vi "dfd_Get NStage VI Description.vi"(6 "nStage nMAC Parameters":T1[](array[typedef]), 7 "multirate filters":T6[](array[typedef]) {"mMRate_SumWl" min=1 max=32 step=1; "mMRate_InputIwl" min=1 max=32 step=1; "mMRate_GainWl" min=1 max=32 step=1; "mMRate_OutputWl" min=1 max=32 step=1; "mMRate_InputWl" min=1 max=32 step=1; "mMRate_CoefWl" min=1 max=32 step=1; "mMRate_Mode" items=["Default"=-1, "No Rate Change"=0, "Interpolation"=1, "Decimation"=2, "Interpolated"=3, "Rational"=4]}, 8 "error in (no error)":errorcluster, 9 "feedback string":string[](array[string]), 10 "M":i32, 11 "L":i32) -> (0 "error out":errorcluster, 3 "NStage VI description":string)   [LabVIEW 2017, in "NI_DigFilterLicensed.lvlib"]
uses:
  <vilib>/addons/Digital Filter Design/NI_DigFilterLicensed.lvlib
  <vilib>/addons/Digital Filter Design/_Objects.llb/DFD Multirate Filter Obj.ctl
  <vilib>/addons/Digital Filter Design/_Objects.llb/DFD Multirate Mode.ctl
  <vilib>/addons/Digital Filter Design/_Objects.llb/DFD Coef Norm Type.ctl
  <vilib>/addons/Digital Filter Design/_Objects.llb/DFD Round-off Mode.ctl
  <vilib>/addons/Digital Filter Design/_Objects.llb/DFD FXP MRate Multiply Mode.ctl
  <vilib>/addons/Digital Filter Design/nMAC.llb/Typedefs/dfd_nMAC_Implementation Parameter.ctl
  <vilib>/addons/Digital Filter Design/nMAC.llb/Typedefs/dfd_nMAC_Execution Mode.ctl
  <vilib>/addons/Digital Filter Design/nMAC.llb/Typedefs/dfd_nMAC_Memory Type.ctl
  <vilib>/addons/Digital Filter Design/nMAC.llb/Typedefs/dfd_nMAC_Coef Reload API.ctl
  <vilib>/addons/Digital Filter Design/nMAC.llb/Typedefs/dfd_nMAC_Coef Map Type.ctl
  <vilib>/addons/Digital Filter Design/NI_DigFilter_CodeGen.lvlib
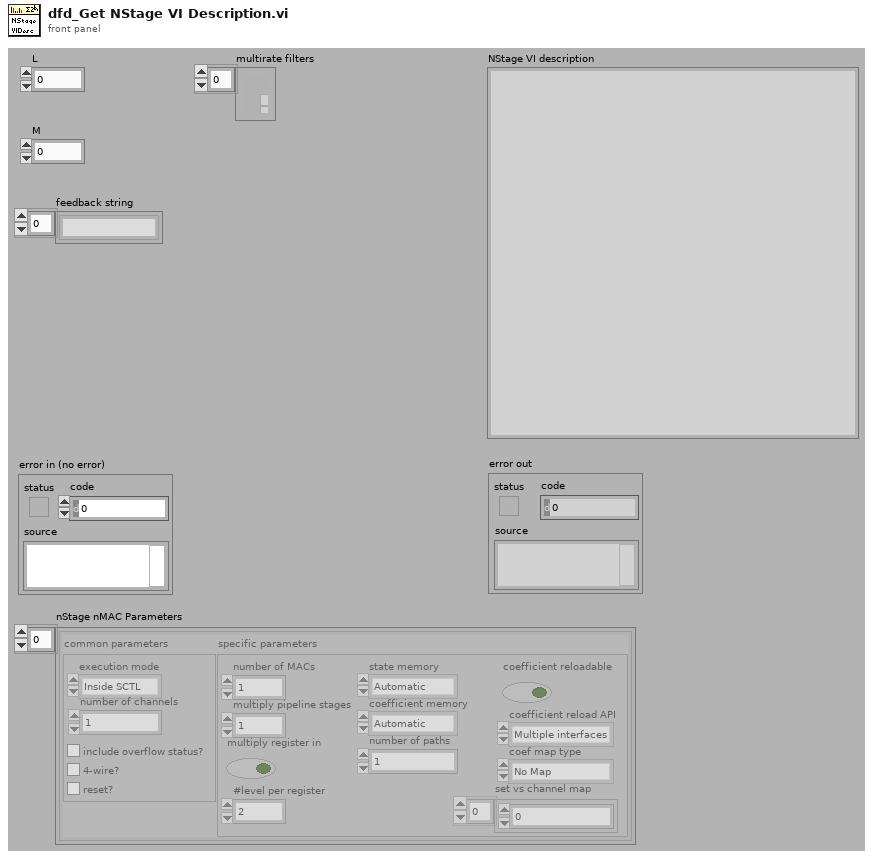
[diagram p1: front panel]
types:
  T1 = typedef "dfd_nMAC_Implementation Parameter.ctl" = cluster{"common parameters":cluster{"execution mode":T2, "number of channels":u32, "reset":bool, "include overflow status":bool, "4-wire":bool}, "specific parameters":cluster{"number of MACs":u32, "multiply pipeline stages":u32, "multiply register in":bool, "#level per register":u32, "state memory":T3, "coefficient memory":T3, "number of paths":u32, "coefficient reloadable":bool, "coefficient reload API":T4, "coef map type":T5, "set vs channel map":u32[]}}
  T2 = typedef "dfd_nMAC_Execution Mode.ctl" = enum16{"Outside SCTL", "Inside SCTL"}
  T3 = typedef "dfd_nMAC_Memory Type.ctl" = enum16{"Automatic", "BRAM", "DRAM"}
  T4 = typedef "dfd_nMAC_Coef Reload API.ctl" = enum16{"Multiple interfaces", "Single interface"}
  T5 = typedef "dfd_nMAC_Coef Map Type.ctl" = enum16{"No Map", "Set Map", "Channel Map"}
  T6 = typedef "NI_DigFilterLicensed.lvlib/DFD Multirate Filter Obj.ctl" = cluster{"mMRate_Structure":enum16{"CIC", "FIR", "IIR", "Lattice"}, "mMRate_Mode":T7, "mMRate_Factor":i32, "mMRate_FIRParams":cluster{"mMRate_FIR_H":dbl[], "mMRate_FIR_IsNyquist?":bool, "mMRate_FIR_IsSymmetric?":bool}, "mMRate_CICParams":cluster{"mMRate_CIC_#Stage":i32, "mMRate_CIC_Lag":i32, "mMRate_CIC_Type":enum16{"Lowpass", "Highpass"}}, "mMRate_Order":i32, "mMRate_Version":string, "mMRate_Comments":string, "mMRate_RationalFactor":cluster{"mMRate_L":i32, "mMRate_M":i32}, "mMRate_Fs":dbl, "mMRate_Quantized?":bool, "mMRate_QFilterGain":dbl, "mMRate_CoefWl":i16, "mMRate_Scaling":cluster{"mMRate_ScaleByPowerOf2?":bool, "mMRate_ScaleType":T8}, "mMRate_InputWl":i16, "mMRate_OutputWl":i16, "mMRate_OutputMode":T9, "mMRate_MultMode":T10, "mMRate_BitPruning":bool, "mMRate_GainWl":i16, "mMRate_OutputFwl":i16, "mMRate_SumIwl":i16, "mMRate_InputIwl ":i16, "mMRate_SumWl":i16, "mMRate_CoefIwl":i16}
  T7 = typedef "NI_DigFilterLicensed.lvlib/DFD Multirate Mode.ctl" = i16
  T8 = typedef "NI_DigFilterLicensed.lvlib/DFD Coef Norm Type.ctl" = enum16{"No Norm", "Time Domain 1-Norm", "Time Domain 2-Norm", "Time Domain Inf-Norm"}
  T9 = typedef "NI_DigFilterLicensed.lvlib/DFD Round-off Mode.ctl" = enum16{"Nearest", "Truncation"}
  T10 = typedef "NI_DigFilterLicensed.lvlib/DFD FXP MRate Multiply Mode.ctl" = enum16{"Truncated", "Full"}
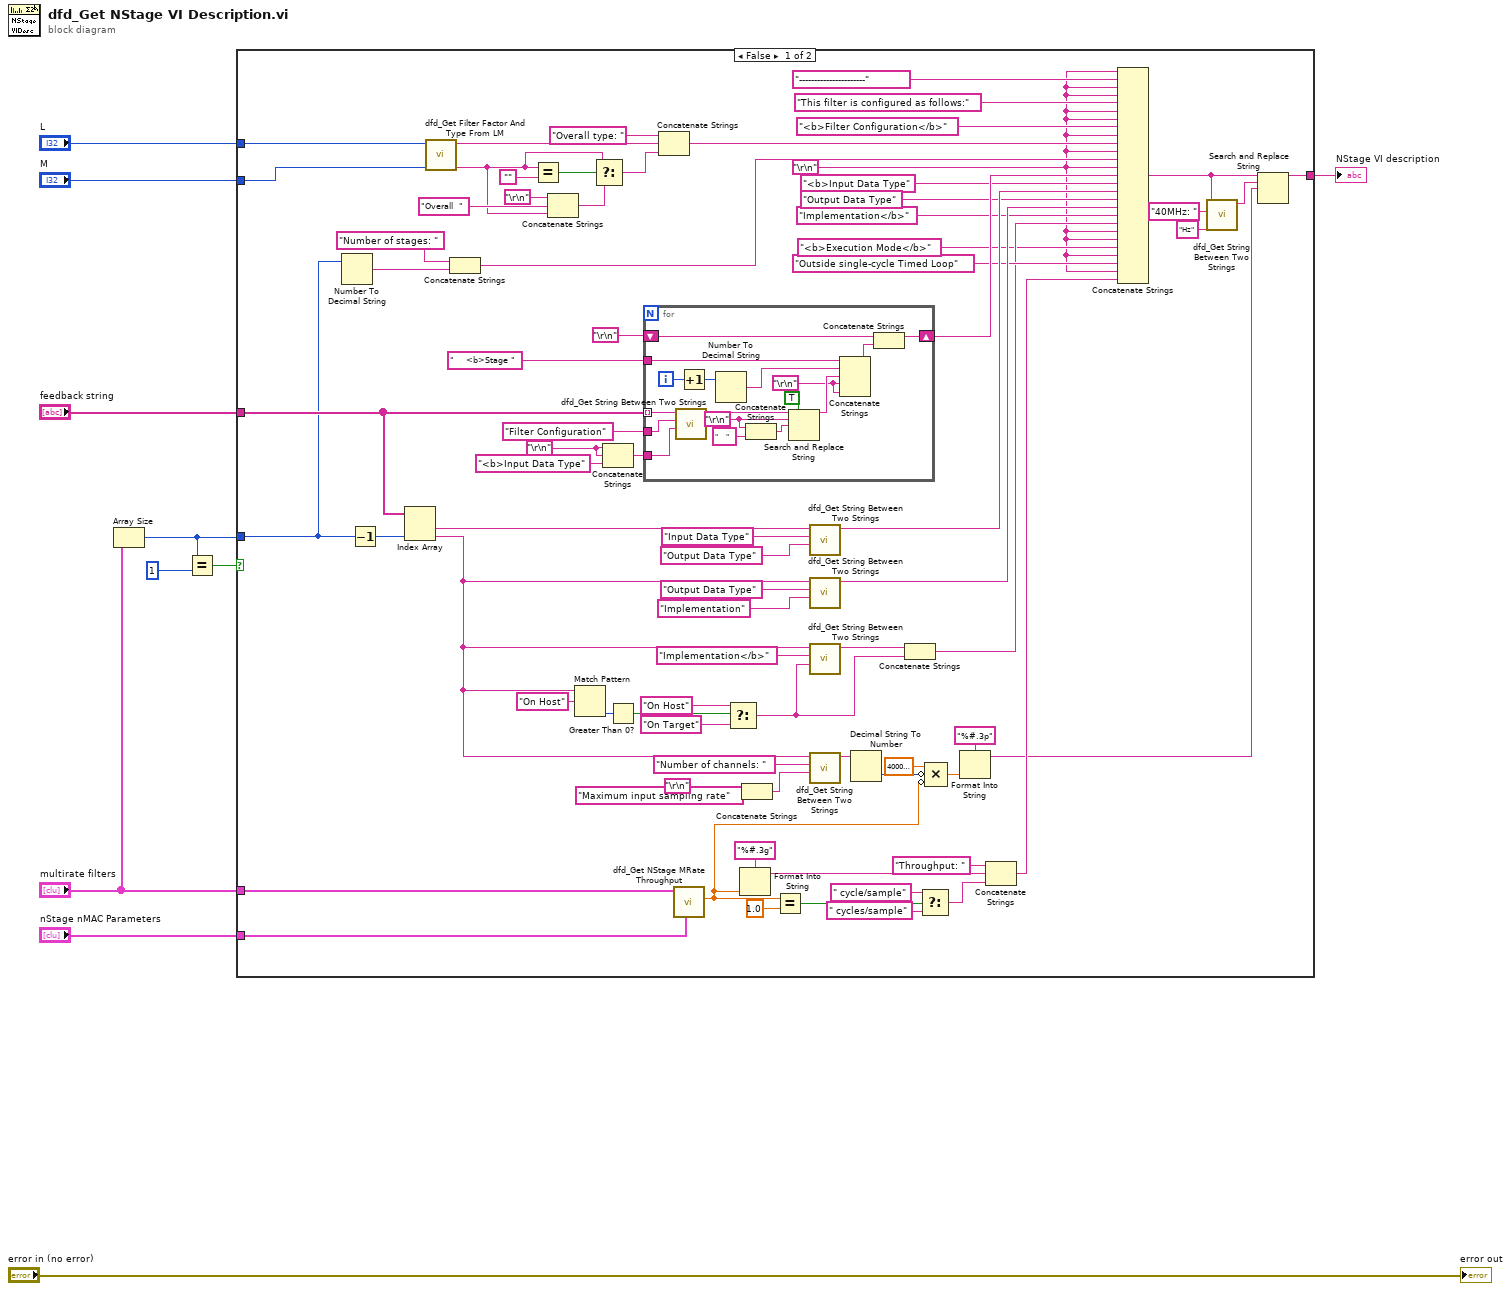
[diagram p0: block diagram]
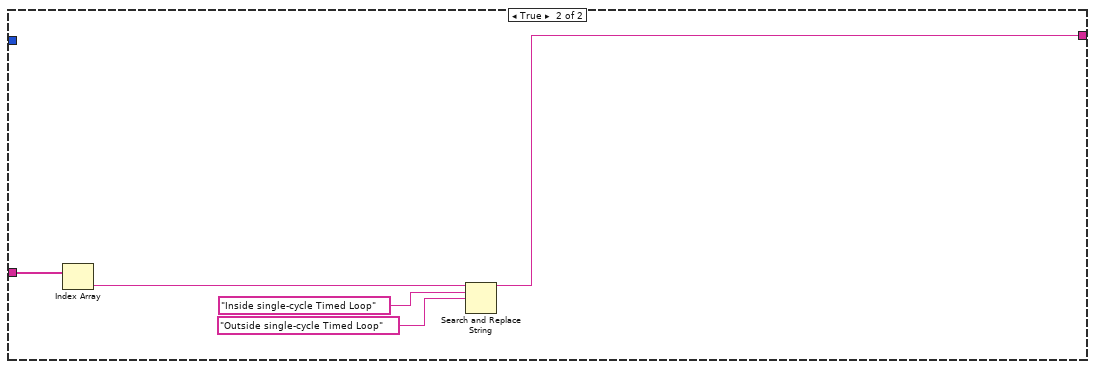
[diagram p2: hidden frame]
diagram:
  n1 = Array Size(array="multirate filters") -> (size(s)=w1:i32)
  n2 = Equal?(x=w1, y=1) -> (x = y?=w8:bool)
  n3 = case shown="False" w8 {
    tunnel: "feedback string" -> [w69 w110]
    tunnel: "L" -> [w82 _]
    tunnel: "M" -> [w81 _]
    tunnel: "multirate filters" -> [w58 _]
    tunnel: [w11 w106] -> w4
    tunnel: "nStage nMAC Parameters" -> [w59 _]
    tunnel: w1 -> [w57 _]
    frame False {
      w31 = "\r\n"
      w61 = "\r\n"
      n4 = Number To Decimal String(number=w57) -> (decimal integer string=w85:string)  [unwired: 1 out]
      n5 = Decrement(x=w57) -> (x-1=w56:i32)
      n6 = Index Array(array=w69, index #2=w56) -> (element #1=w55:string, element #2=w26:string)  [unwired: 1 in]
      n7 = call <vilib>:"dfd_Get Filter Factor And Type From LM.vi"("M"=w81, "L"=w82) -> ("Factor"=w74:string, "Type"=w80:string)  [unwired: 8 out]
      n8 = Concatenate Strings("Number of stages: " ("string"), w85) -> (w83:string)
      n9 = Equal?(x=w74, y="") -> (x = y?=w77:bool)
      n10 = Concatenate Strings("\r\n", "Overall  " ("string"), w74) -> (w73:string)
      n11 = Match Pattern(string=w26, regular expression="On Host") -> (offset past match=w44:i32)  [unwired: 4 out]
      n12 = Select(t=w74, s=w77, f=w73) -> (s? t:f=w72:string)
      n13 = Concatenate Strings(w61, w61, "<b>Input Data Type" ("Begin String")) -> (w86:string)
      n14 = Greater Than 0?(x=w44) -> (x > 0?=w38:bool)
      n15 = for {
        tunnel: w69 -> [w105] mode=indexing
        tunnel: "Filter Configuration" ("Begin String") -> [w104]
        tunnel: w86 -> [w103]
        tunnel: "    <b>Stage " ("Begin String") -> [w99]
        shift-right: [w94] -> w70
        shift-left: "\r\n" -> [w93]
        i -> [w102]
        w89 = "\r\n"
        w97 = "\r\n"
        n16 = call <vilib>:"dfd_Get String Between Two Strings.vi"("End String"=w103, "Begin String"=w104, "Source String"=w105) -> ("Output String"=w98:string)  [unwired: 8 out]
        n17 = Increment(x=w102) -> (x+1=w101:i32)
        n18 = Number To Decimal String(number=w101) -> (decimal integer string=w100:string)  [unwired: 1 out]
        n19 = Concatenate Strings(w97, "    " ("string")) -> (w96:string)
        n20 = Search and Replace String(replace all?=TRUE ("replace all? (F)"), input string=w98, search string=w97, replace string=w96) -> (result string=w95:string)  [unwired: 1 in, 6 out]
        n21 = Concatenate Strings(w99, w100, w95, w89, w89) -> (w92:string)
        n22 = Concatenate Strings(w93, w92) -> (w94:string)
      }
      n23 = Concatenate Strings("Overall type: " ("string"), w80, w72) -> (w71:string)
      n24 = call <vilib>:"dfd_Get NStage MRate Throughput.vi"("nStage nMAC Parameters"=w59, "multirate filters"=w58) -> ("throughput"=w17:dbl)  [unwired: 1 in, 8 out]
      n25 = Select(t="On Host" ("regular expression"), s=w38, f="On Target") -> (s? t:f=w34:string)
      n26 = Format Into String(format string="%#.3g", w17) -> (resulting string=w28:string)  [unwired: 2 in, 1 out]
      n27 = Concatenate Strings("\r\n", "Maximum input sampling rate" ("string")) -> (w23:string)
      n28 = Equal?(x=w17, y=1.0) -> (x = y?=w67:bool)
      n29 = call <vilib>:"dfd_Get String Between Two Strings.vi"("End String"="Output Data Type", "Begin String"="Input Data Type", "Source String"=w55) -> ("Output String"=w50:string)  [unwired: 8 out]
      n30 = call <vilib>:"dfd_Get String Between Two Strings.vi"("End String"="Implementation", "Begin String"="Output Data Type", "Source String"=w26) -> ("Output String"=w46:string)  [unwired: 8 out]
      n31 = call <vilib>:"dfd_Get String Between Two Strings.vi"("End String"=w34, "Begin String"="Implementation</b>", "Source String"=w26) -> ("Output String"=w35:string)  [unwired: 8 out]
      n32 = call <vilib>:"dfd_Get String Between Two Strings.vi"("End String"=w23, "Begin String"="Number of channels: " ("Source String"), "Source String"=w26) -> ("Output String"=w22:string)  [unwired: 8 out]
      n33 = Decimal String To Number(string=w22) -> (number=w18:i32)  [unwired: 3 out]
      n34 = Concatenate Strings(w35, w34) -> (w33:string)
      n35 = Select(t=" cycle/sample" ("decimal integer string"), s=w67, f=" cycles/sample" ("decimal integer string")) -> (s? t:f=w64:string)
      n36 = Compound Arithmetic op=MULTIPLY(40000000.0, invert w18, invert w17) -> (w19:dbl)
      n37 = Format Into String(format string="%#.3p", w19) -> (resulting string=w12:string)  [unwired: 2 in, 1 out]
      n38 = Concatenate Strings("Throughput: " ("string"), w28, w64) -> (w41:string)
      n39 = Concatenate Strings(w31, "----------------------", w31, w31, "This filter is configured as follows:", w31, w31, "<b>Filter Configuration</b>", w31, w71, w31, w83, w31, w70, "<b>Input Data Type", w50, "Output Data Type", w46, "Implementation</b>", w33, w31, w31, "<b>Execution Mode</b>", w31, "Outside single-cycle Timed Loop" ("string"), w31, w41) -> (w14:string)
      n40 = call <vilib>:"dfd_Get String Between Two Strings.vi"("End String"="Hz", "Begin String"="40MHz: ", "Source String"=w14) -> ("Output String"=w13:string)  [unwired: 8 out]
      n41 = Search and Replace String(input string=w14, search string=w13, replace string=w12) -> (result string=w11:string)  [unwired: 1 in, 7 out]
    }
    frame True {
      n42 = Index Array(array=w110) -> (element=w109:string)  [unwired: 1 in]
      n43 = Search and Replace String(input string=w109, search string="Inside single-cycle Timed Loop", replace string="Outside single-cycle Timed Loop" ("replace string (\"\")")) -> (result string=w106:string)  [unwired: 1 in, 7 out]
    }
  }
  "NStage VI description" <- w4
  "error out" <- "error in (no error)"
